vi "Configure.vi"(8 "error in":errorcluster, 10 "name":string, 11 "PAS in":refnum<class "PAS.lvclass">) -> (0 "error out":errorcluster, 3 "PAS out":refnum<class "PAS.lvclass">)   [LabVIEW 2015, in "PAS.lvclass"]
doc: "Configure the Instrument object. The default behavior is to provide a name and define a command enqueuer."
uses:
  PAS.lvclass
  Switch/Switch.lvclass
  Instrument/Instrument.lvclass/Instrument.ctl
  PAS.lvclass/PAS.ctl
  File IO/Class/File Observer.lvclass/File Observer.ctl
  Switch/Switch.lvclass/Switch.ctl
  Instrument/Read Cfg Session.vi
  Switch/Write LastSwitch.vi
  File IO/Class/Accessors/Write File Ext.vi
  File IO/Class/Accessors/Write File Prefix.vi
  File IO/Class/Accessors/Write Max Size.vi
  File IO/Class/Write SwitchonSize_.vi
  File IO/Class/Accessors/Write Top Data Path.vi
  File IO/Class/Write Write.vi
  Read Data.vi
  Read Cells.vi
  Data/Main/Read CellData.vi
  <vilib>/Utility/config.llb/Read Key (Double).vi
  <vilib>/Utility/config.llb/Read Key (Boolean).vi
  <vilib>/Utility/config.llb/Read Key (I32).vi
  <vilib>/Utility/config.llb/Read Key (String).vi
  Switch/Write maxElapseTime.vi
  Cell/Write extParams.vi
  Data/Main/Write CellData.vi
  Write Cells.vi
  Write Data.vi
  Instrument/Instrument.lvclass
  <userlib>/_Session Fwk/Session - Root.lvclass
  Data/Main/PAS Data.lvclass
  Cell/PAS Cell.lvclass
  Data/Cell/PAS Cell Data.lvclass
  File IO/Class/File Observer.lvclass
  Session APIs/File Access/Config Data/Config Data.lvclass
  <vilib>/Utility/config.llb/NI_LVConfig.lvlib
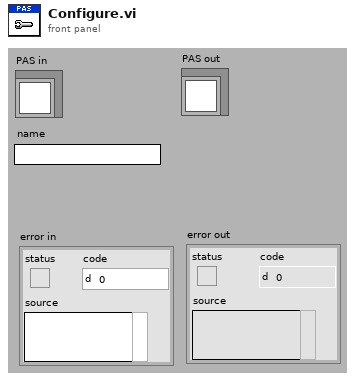
[diagram p1: front panel]
types:
  T1 = typedef "Session - Root.lvclass/Session Handle.ctl" = refnum<data-value>
  T2 = typedef "NI_LVConfig.lvlib/Config Data RefNum.ctl" = refnum<k1>
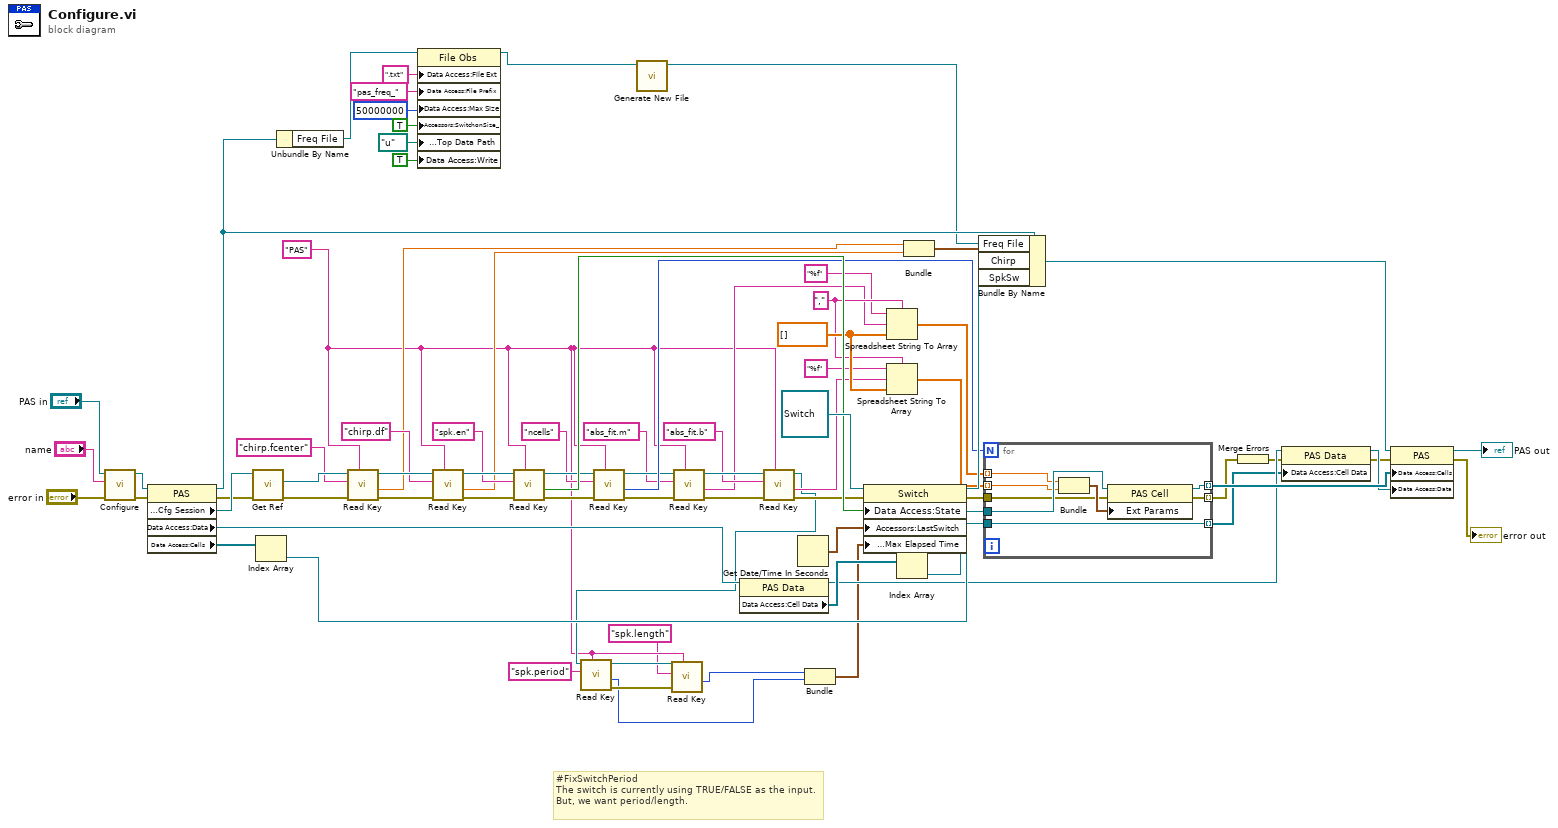
[diagram p0: block diagram]
diagram:
  w33 = dbl[] []
  w32 = "," ("delimiter (Tab)")
  w17 = "PAS" ("section")
  # "#FixSwitchPeriod\nThe switch is currently using TRUE/FALSE as the input.  But, we want period/length."
  n1 = call-parent "Configure.vi"("error in"="error in", "name"="name", "Instrument in"="PAS in") -> ("error out"=w73:errorcluster, "Instrument out"=w74:refnum<class "PAS.lvclass">)  [unwired: 7 in]
  n2 = property class="PAS"(reference=w74, error in=w73) -> (reference out=w10:refnum<class "PAS.lvclass">, error out=w71:errorcluster, "Accessors:Cfg Session"=w72:T1, "Data Access:Data"=w50:refnum<class "PAS Data.lvclass">, "Data Access:Cells"=w45:refnum<class "PAS Cell.lvclass">[])
  n3 = call "Get Ref.vi"("error in"=w71, "Session Handle In"=w72) -> ("error out"=w69:errorcluster, "Ref"=w70:T2)  [unwired: 7 in, 1 out]
  n4 = Index Array(array=w45) -> (element=w44:refnum<class "PAS Cell.lvclass">)  [unwired: 1 in]
  n5 = Unbundle By Name(w10) -> ("Freq File"=w9:refnum<class "File Observer.lvclass">)
  n6 = call-poly <vilib>:"Read Key.vi"("section"=w17, "error in (no error)"=w69, "key"="chirp.fcenter", "refnum"=w70) -> ("error out"=w66:errorcluster, "value"=w61:dbl, "refnum out"=w67:T2)  [unwired: 4 in, 1 out]
  n7 = property class="File Obs"(reference=w9, "Data Access:File Ext"=".txt" ("File Ext"), "Data Access:File Prefix"="pas_freq_" ("File Prefix"), "Data Access:Max Size"=i64 50000000 ("Max Size"), "Accessors:SwitchonSize_"=TRUE ("SwitchonSize_"), "Data Access:Top Data Path"=path "u:/" ("Top Data Path"), "Data Access:Write"=TRUE ("Write")) -> (reference out=w2:refnum<class "File Observer.lvclass">)  [unwired: 1 in, 1 out]
  n8 = call-poly <vilib>:"Read Key.vi"("section"=w17, "error in (no error)"=w66, "key"="chirp.df", "refnum"=w67) -> ("error out"=w63:errorcluster, "value"=w60:dbl, "refnum out"=w64:T2)  [unwired: 4 in, 1 out]
  n9 = call-poly <vilib>:"Read Key.vi"("section"=w17, "error in (no error)"=w63, "key"="spk.en", "refnum"=w64) -> ("error out"=w54:errorcluster, "value"=w57:bool, "refnum out"=w53:T2)  [unwired: 4 in, 1 out]
  n10 = call-poly <vilib>:"Read Key.vi"("section"=w17, "error in (no error)"=w54, "key"="ncells", "refnum"=w53) -> ("error out"=w38:errorcluster, "value"=w51:i32, "refnum out"=w39:T2)  [unwired: 4 in, 1 out]
  n11 = call-dynamic "Generate New File.vi"("File Obs in"=w2) -> ("File Obs out"=w1:refnum<class "File Observer.lvclass">)  [unwired: 8 in, 2 out]
  n12 = call-poly <vilib>:"Read Key.vi"("section"=w17, "error in (no error)"=w38, "key"="abs_fit.m", "refnum"=w39) -> ("error out"=w35:errorcluster, "value"=w22:string, "refnum out"=w36:T2)  [unwired: 4 in, 1 out]
  n13 = property class="PAS Data"(reference=w50) -> (reference out=w42:refnum<class "PAS Data.lvclass">, "Data Access:Cell Data"=w49:refnum<class "PAS Cell Data.lvclass">[])  [unwired: 1 in, 1 out]
  n14 = call-poly <vilib>:"Read Key.vi"("section"=w17, "error in (no error)"=w35, "key"="abs_fit.b", "refnum"=w36) -> ("error out"=w31:errorcluster, "value"=w23:string, "refnum out"=w19:T2)  [unwired: 4 in, 1 out]
  n15 = call-poly <vilib>:"Read Key.vi"("section"=w17, "key"="spk.period", "refnum"=w19) -> ("error out"=w14:errorcluster, "value"=w13:i32, "refnum out"=w18:T2)  [unwired: 5 in, 1 out]
  n16 = call-poly <vilib>:"Read Key.vi"("section"=w17, "error in (no error)"=w14, "key"="spk.length", "refnum"=w18) -> ("value"=w12:i32)  [unwired: 4 in, 3 out]
  n17 = Get Date/Time In Seconds() -> (seconds since 1Jan1904=w56:timestamp)
  n18 = Bundle("value"=w12, "value"=w13) -> (w11:cluster{"value":i32, "value":i32})  [unwired: 1 in]
  n19 = property class="Switch"(reference=refnum<class "Switch.lvclass"> refnum ("SpkSw"), error in=w31, "Data Access:State"=w57, "Accessors:LastSwitch"=w56, "Data Access:Max Elapsed Time"=w11) -> (reference out=w55:refnum<class "Switch.lvclass">, error out=w28:errorcluster)
  n20 = Spreadsheet String To Array(delimiter (Tab)=w32, format string="%f", spreadsheet string=w22, array type (2D Dbl)=w33) -> (array=w30:dbl[])
  n21 = Spreadsheet String To Array(delimiter (Tab)=w32, format string="%f", spreadsheet string=w23, array type (2D Dbl)=w33) -> (array=w29:dbl[])
  n22 = Index Array(array=w49) -> (element=w48:refnum<class "PAS Cell Data.lvclass">)  [unwired: 1 in]
  n23 = Bundle("value"=w61, "value"=w60) -> (w59:cluster{"value":dbl, "value":dbl})  [unwired: 1 in]
  n24 = Bundle By Name(cluster=w10, "Freq File"=w1, "Chirp"=w59, "SpkSw"=w55) -> (w47:refnum<class "PAS.lvclass">)
  n25 = for {
    N: w51 -> [_]
    tunnel: w48 -> [w85]
    tunnel: [w85] -> w41 mode=indexing
    tunnel: w44 -> [w83]
    tunnel: [w84] -> w43 mode=indexing
    tunnel: w30 -> [w82] mode=indexing
    tunnel: w29 -> [w81] mode=indexing
    tunnel: w28 -> [w79]
    tunnel: [w78] -> w27 mode=indexing
    n26 = Bundle(w82, w81) -> (w80:cluster{dbl, dbl})  [unwired: 1 in]
    n27 = property class="PAS Cell"(reference=w83, error in=w79, "Ext Params"=w80) -> (reference out=w84:refnum<class "PAS Cell.lvclass">, error out=w78:errorcluster)
  }
  n28 = Merge Errors(w27) -> (w26:errorcluster)
  n29 = property class="PAS Data"(reference=w42, error in=w26, "Data Access:Cell Data"=w41) -> (reference out=w40:refnum<class "PAS Data.lvclass">, error out=w25:errorcluster)
  n30 = property class="PAS"(reference=w47, error in=w25, "Data Access:Cells"=w43, "Data Access:Data"=w40) -> (reference out=→"PAS out":refnum<class "PAS.lvclass">, error out=→"error out":errorcluster)
